vi "macro_SwerveModStateNew4.vi"   [LabVIEW 2019, in "Trajectory_Library.lvlib"]
uses:
  Conv_Deg_Radians.vi
  Rotation2d_CreateAngle.vi
  Trajectory_Library.lvlib
types:
  T1 = typedef "Trajectory_Library.lvlib/ROTATION2D.ctl" = cluster{"VALUE":dbl, "COS":dbl, "SIN":dbl}
  T2 = typedef "Trajectory_Library.lvlib/SWERVE_DRIVE_MODULE_STATE.ctl" = cluster{"Speed":dbl, "Angle":T1}
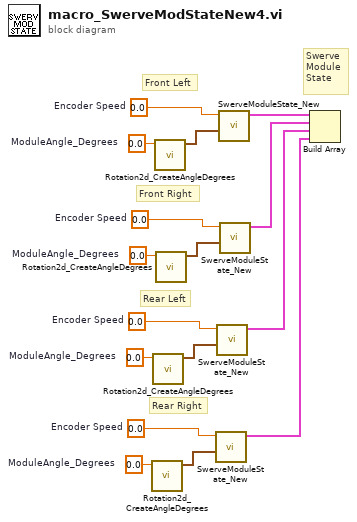
[diagram p0: block diagram]
diagram:
  w4 = 0.0  # ModuleAngle_Degrees
  w6 = 0.0  # Encoder Speed
  w7 = 0.0  # ModuleAngle_Degrees
  w9 = 0.0  # Encoder Speed
  w10 = 0.0  # ModuleAngle_Degrees
  w12 = 0.0  # Encoder Speed
  w14 = 0.0  # ModuleAngle_Degrees
  w16 = 0.0  # Encoder Speed
  # "Front Left"
  # "Swerve\nModule\nState"
  # "Rear Right"
  # "Rear Left"
  # "Front Right"
  n1 = call "Rotation2d_CreateAngleDegrees.vi"("Angle_Degrees"=w4) -> ("ROTATION"=w5:T1)  [unwired: 10 in]
  n2 = call "Rotation2d_CreateAngleDegrees.vi"("Angle_Degrees"=w7) -> ("ROTATION"=w8:T1)  [unwired: 10 in]
  n3 = call "Rotation2d_CreateAngleDegrees.vi"("Angle_Degrees"=w14) -> ("ROTATION"=w15:T1)  [unwired: 10 in]
  n4 = call "Rotation2d_CreateAngleDegrees.vi"("Angle_Degrees"=w10) -> ("ROTATION"=w11:T1)  [unwired: 10 in]
  n5 = call "SwerveModuleState_New.vi"("ROTATION"=w5, "Speed"=w6) -> ("SWERVE_DRIVE_MODULE_STATE"=w1:T2)  [unwired: 9 in]
  n6 = call "SwerveModuleState_New.vi"("ROTATION"=w8, "Speed"=w9) -> ("SWERVE_DRIVE_MODULE_STATE"=w2:T2)  [unwired: 9 in]
  n7 = call "SwerveModuleState_New.vi"("ROTATION"=w15, "Speed"=w16) -> ("SWERVE_DRIVE_MODULE_STATE"=w13:T2)  [unwired: 9 in]
  n8 = call "SwerveModuleState_New.vi"("ROTATION"=w11, "Speed"=w12) -> ("SWERVE_DRIVE_MODULE_STATE"=w3:T2)  [unwired: 9 in]
  n9 = Build Array(w13, w3, w2, w1) -> ()  [unwired: 1 out]
